vi "Update.vi"(8 "error in (no error)":errorcluster, 10 "Message in":refnum<class "UpdateMessage.lvclass">, 11 "Cascade in":refnum<class "Cascade.lvclass">) -> (0 "error out":errorcluster, 3 "Cascade out":refnum<class "Cascade.lvclass">)   [LabVIEW 2012, in "Cascade.lvclass"]
doc: "The update method processes the command 'update'. \n\nThe command 'update' is used for receiving new values to be set to the private data of the class. This could be seen as a public set method for setting new parameters to the private class data."
uses:
  Cascade.lvclass
  <vilib>/Distrio/Murmex/UpdateMessage/UpdateMessage.lvclass
  Cascade.lvclass/Cascade.ctl
  <vilib>/Distrio/Murmex/Murmex/Murmex.lvclass
panel:
  # "This method is called when the UPDATE\ntrigger is sent. \n\nOverride this method when your component needs to\nrespond to this trigger. \n\nCall parent for proper implementation"
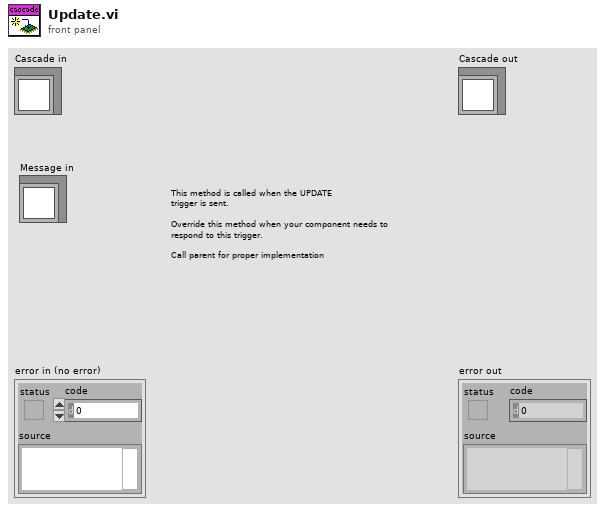
[diagram p1: front panel]
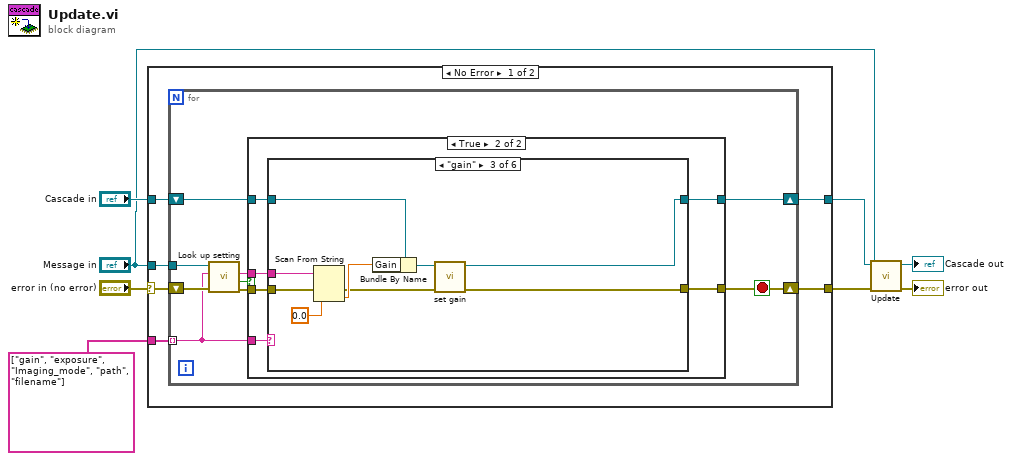
[diagram p0: block diagram]
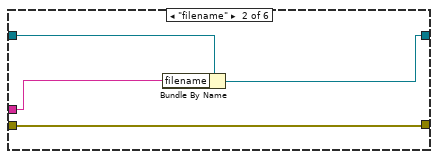
[diagram p4: hidden frame]
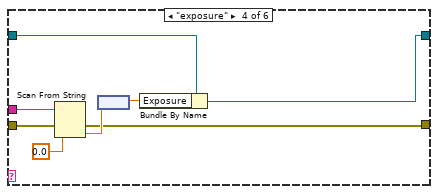
[diagram p5: hidden frame]
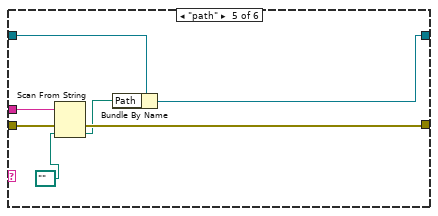
[diagram p6: hidden frame]
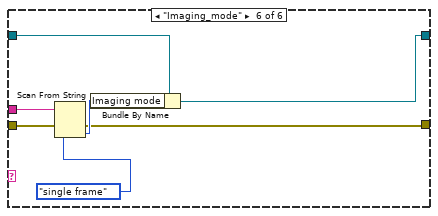
[diagram p7: hidden frame]
diagram:
  n1 = case shown="No Error" "error in (no error)" {
    selector: "error in (no error)" -> [w14 w70]
    tunnel: "Cascade in" -> [w13 w69]
    tunnel: "Message in" -> [w12 _]
    tunnel: string[] ["gain", "exposure", "Imaging_mode", "path", "filename"] -> [w11 _]
    tunnel: [w10 w70] -> w2
    tunnel: [w9 w69] -> w1
    frame No Error {
      n2 = for {
        shift-right: [w15] -> w10
        shift-left: w14 -> [w23]
        shift-right: [w16] -> w9
        shift-left: w13 -> [w18]
        tunnel: w12 -> [w22]
        tunnel: w11 -> [w20] mode=indexing
        stop <- w15 stop-if-true
        n3 = call <vilib>:"Look up setting.vi"("error in (no error)"=w23, "tag name"=w20, "UpdateMessage in"=w22) -> ("error out"=w17:errorcluster, "found?"=w21:bool, "value"=w19:string)  [unwired: 5 in, 1 out]
        n4 = case shown="True" w21 {
          tunnel: w20 -> [_ w31]
          tunnel: w19 -> [_ w29]
          tunnel: w18 -> [w25 w28]
          tunnel: w17 -> [w24 w30]
          tunnel: [w24 w27] -> w15
          tunnel: [w25 w26] -> w16
          frame False {
          }
          frame True {
            n5 = case shown="\"gain\"" w31 {
              tunnel: w30 -> [w33 w35 w46 w54 w61 w68]
              tunnel: w29 -> [_ w34 w45 w53 w60 w67]
              tunnel: w28 -> [w32 w37 w44 w52 w59 w66]
              tunnel: [w33 w35 w40 w48 w57 w63] -> w27
              tunnel: [w32 w36 w38 w49 w58 w64] -> w26
              frame Default {
              }
              frame "filename" {
                n6 = Bundle By Name(cluster=w37, "filename"=w34) -> (w36:refnum<class "Cascade.lvclass">)
              }
              frame "gain" {
                n7 = Scan From String(input string=w45, error in=w46, default 1=0.0 ("settings.Gain")) -> (error out=w41:errorcluster, output 1=w43:dbl)  [unwired: 2 in, 2 out]
                n8 = Bundle By Name(cluster=w44, "Gain"=w43) -> (w39:refnum<class "Cascade.lvclass">)
                n9 = call-dynamic "set gain.vi"("error in (no error)"=w41, "Cascade in"=w39) -> ("error out"=w40:errorcluster, "Cascade out"=w38:refnum<class "Cascade.lvclass">)  [unwired: 8 in]
              }
              frame "exposure" {
                n10 = Scan From String(input string=w53, error in=w54, default 1=0.0 ("settings.Gain")) -> (error out=w48:errorcluster, output 1=w51:dbl)  [unwired: 2 in, 2 out]
                n11 = node(w51) -> (w47:dbl[unit])
                n12 = Bundle By Name(cluster=w52, "Exposure"=w47) -> (w49:refnum<class "Cascade.lvclass">)
              }
              frame "path" {
                n13 = Scan From String(input string=w60, error in=w61, default 1=path "" ("settings.Path")) -> (error out=w57:errorcluster, output 1=w55:path)  [unwired: 2 in, 2 out]
                n14 = Bundle By Name(cluster=w59, "Path"=w55) -> (w58:refnum<class "Cascade.lvclass">)
              }
              frame "Imaging_mode" {
                n15 = Scan From String(input string=w67, error in=w68, default 1=enum16{"single frame", "free run mode"}."single frame" ("settings.Imaging mode")) -> (error out=w63:errorcluster, output 1=w65:enum16{"single frame", "free run mode"})  [unwired: 2 in, 2 out]
                n16 = Bundle By Name(cluster=w66, "Imaging mode"=w65) -> (w64:refnum<class "Cascade.lvclass">)
              }
            }
          }
        }
      }
    }
    frame Error {
    }
  }
  n17 = call-parent "Update.vi"("error in (no error)"=w2, "Message in"="Message in", "Murmex in"=w1) -> ("error out"=→"error out":errorcluster, "Murmex out"=→"Cascade out":refnum<class "Cascade.lvclass">)  [unwired: 7 in]
